vi "SP Find Limit by Format.vi"(8 "Limit Format":T3, 10 "Parameter":T1={"Stimulus Port"=1, "Response Port"=1} caption="Parameter String" {"Stimulus Port" min=1 step=1; "Response Port" min=1 step=1}, 11 "Limits":T2[](array[typedef]) {"Parameter"."Stimulus Port" min=1 step=1; "Parameter"."Response Port" min=1 step=1}) -> (0 "Found?":bool, 3 "Limits":T2[](array[typedef]) {"Parameter"."Stimulus Port" min=1 step=1; "Parameter"."Response Port" min=1 step=1})   [LabVIEW 2011]
uses:
  TypeDefs/SP Limit.ctl
  TypeDefs/SP Parameter.ctl
  TypeDefs/SP Format.ctl
  TypeDefs/SP Limit Type.ctl
  TypeDefs/SP Limit Point.ctl
  Test Referential Limit.ctl
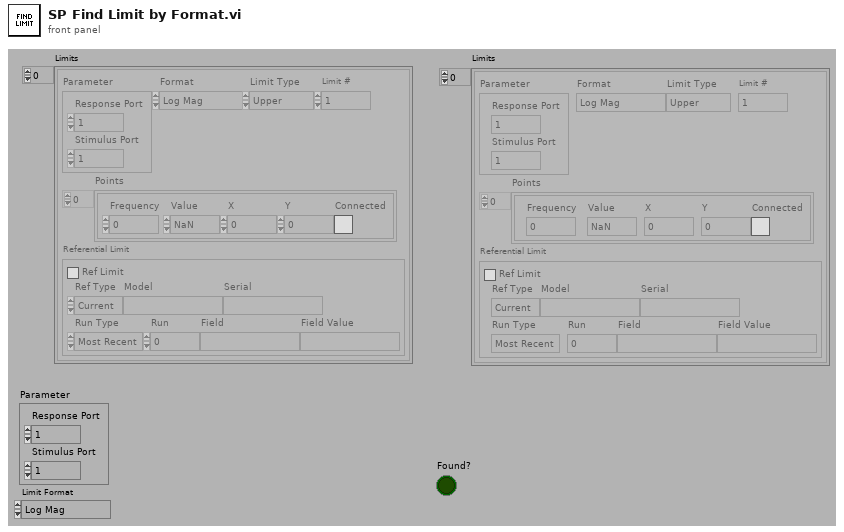
[diagram p1: front panel]
types:
  T1 = typedef "SP Parameter.ctl" = cluster{"Stimulus Port":i8, "Response Port":i8}
  T2 = typedef "SP Limit.ctl" = cluster{"Parameter":T1, "Format":T3, "Limit Type":T4, "Points":T5[], "Referential Limit":T6, "Limit #":i8}
  T3 = typedef "SP Format.ctl" = enum16{"Log Mag", "Lin Mag", "SWR", "Phase", "Expanded Phase", "Delay", "Insertion Loss", "Isolation", "Return Loss"}
  T4 = typedef "SP Limit Type.ctl" = enum16{"Upper", "Lower", "Delta", "Filter", "Referential"}
  T5 = typedef "SP Limit Point.ctl" = cluster{"Frequency":dbl, "Value":dbl, "X":dbl, "Y":dbl, "Connected":bool}
  T6 = typedef "Test Referential Limit.ctl" = cluster{"Ref Limit":bool, "Ref Type":enum16{"Current", "Specify"}, "Model":string, "Serial":string, "Run Type":enum16{"Most Recent", "Run #", "Match Field"}, "Run":i32, "Field":string, "Field Value":string}
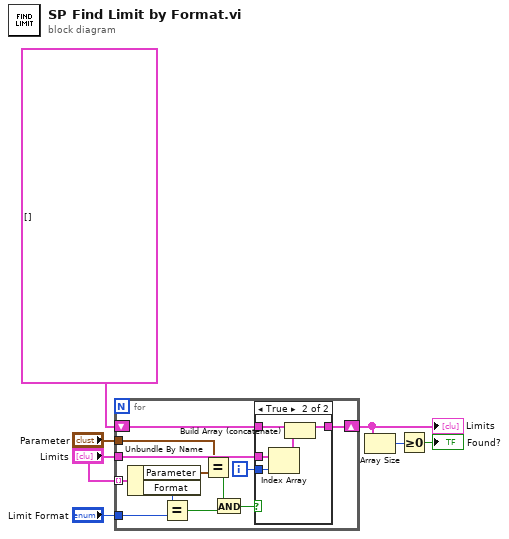
[diagram p0: block diagram]
diagram:
  n1 = for {
    tunnel: "Limits" -> [w19] mode=indexing
    tunnel: "Limits" -> [w18]
    tunnel: "Limit Format" -> [w16]
    shift-right: [w13] -> w4
    shift-left: T2[] [] ("Limits") -> [w14]
    tunnel: "Parameter" -> [w10]
    i -> [w15]
    n2 = Unbundle By Name(w19) -> ("Parameter"=w11:T1, "Format"=w17:T3)
    n3 = Equal?(x=w17, y=w16) -> (x = y?=w12:bool)
    n4 = Equal?(x=w10, y=w11) -> (x = y?=w9:bool)
    n5 = And(x=w9, y=w12) -> (x .and. y?=w8:bool)
    n6 = case shown="True" w8 {
      tunnel: w18 -> [_ w25]
      tunnel: w15 -> [_ w24]
      tunnel: w14 -> [w20 w22]
      tunnel: [w20 w21] -> w13
      frame False {
      }
      frame True {
        n7 = Index Array(array=w25, index=w24) -> (element=w23:T2)
        n8 = Build Array (concatenate)(w22, w23) -> (w21:T2[])
      }
    }
  }
  "Limits" <- w4
  n9 = Array Size(array=w4) -> (size(s)=w3:i32)
  n10 = Greater Or Equal To 0?(x=w3) -> (x >= 0?=→"Found?":bool)
